vi "Handle Last Ack Core.vi"(4 "error in (no error)":errorcluster, 6 "Last Ack":refnum<class "Last Ack.lvclass">, 7 "Publisher in":refnum<class "Publisher.lvclass">) -> (0 "error out":errorcluster, 3 "Publisher out":refnum<class "Publisher.lvclass">)   [LabVIEW 2020, in "Publisher.lvlib" / "Publisher.lvclass"]
doc: "(<B>Filename</B>: Actor Framework.lvlib:Actor.lvclass:Handle Last Ack Core.vi)\n\nDefines how the caller actor responds to the Last Ack message from a nested actor. The Last Ack message is the final message a nested actor sends to its caller before it shuts down. The message contains information about the final state of the nested actor.\n\nThis implementation removes the stopped actor from the enqueuer and actor look up tables."
uses:
  Publisher.lvclass
  PPL/HDH.Actor Framework.Core.Actor.lvlibp/1abvi3w/vi.lib/ActorFramework/LastAck/Last Ack.lvclass
  Publisher.lvclass/Publisher.ctl
  PPL/HDH.Actor Framework.Core.Actor.lvlibp/1abvi3w/vi.lib/ActorFramework/Message Enqueuer/Message Enqueuer.lvclass
  PPL/HDH.Actor Framework.Core.Actor.lvlibp/1abvi3w/vi.lib/ActorFramework/Actor/Actor.lvclass
  PPL/HDH.Data.Generic.lvlibp
  PPL/HDH.Actor Framework.Core.Utility.lvlibp
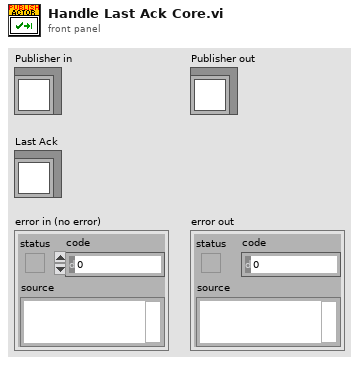
[diagram p1: front panel]
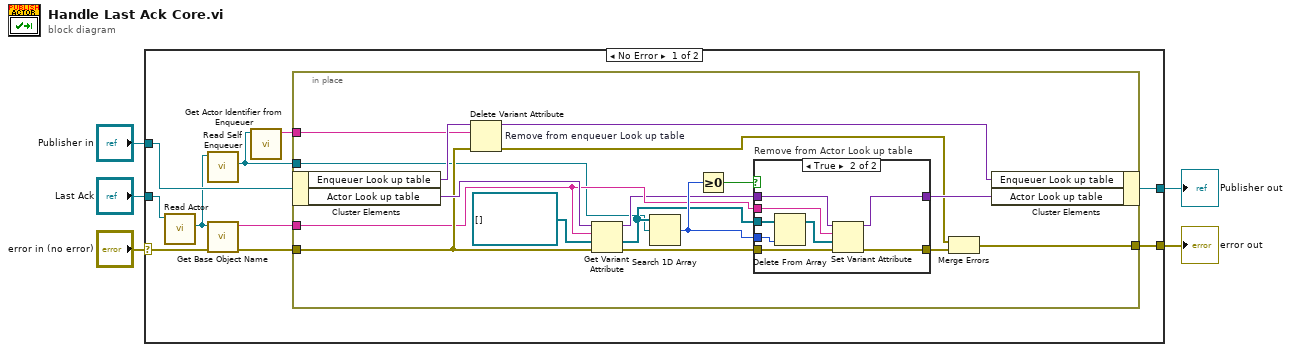
[diagram p0: block diagram]
diagram:
  n1 = case shown="No Error" "error in (no error)" {
    selector: "error in (no error)" -> [w10 w44]
    tunnel: [w8 w44] -> w4
    tunnel: [w7 w43] -> w3
    tunnel: "Publisher in" -> [w15 w43]
    tunnel: "Last Ack" -> [w13 _]
    frame No Error {
      n2 = call "Read Actor.vi"("Last Ack"=w13) -> ("Actor"=w12:refnum<class "Actor.lvclass">)  [unwired: 10 in]
      n3 = call "Read Self Enqueuer.vi"("Actor"=w12) -> ("Self Enqueuer"=w6:refnum<class "Message Enqueuer.lvclass">)  [unwired: 10 in]
      n4 = call "Get Base Object Name.vi"("error in (no error)"=w10, "Object in"=w12) -> ("error out"=w9:errorcluster, "Base class name"=w11:string)  [unwired: 8 in]
      n5 = call "Get Actor Identifier from Enqueuer.vi"("Message Enqueuer in"=w6) -> ("Actor ID string out"=w14:string)  [unwired: 9 in, 1 out]
      n6 = in-place {
        in-place-border: w14 -> [w27]
        in-place-border: w11 -> [w23]
        in-place-border: w9 -> [w28]
        in-place-border: [w17] -> w8
        in-place-border: w6 -> [w16]
        n7 = in-place-cluster #1(w15) -> ("Enqueuer Look up table"=w29:variant, "Actor Look up table"=w31:variant)
        n8 = Delete Variant Attribute "Remove from enqueuer Look up table"(4:w28, 6:w27, 7:w29) -> (0:w19:errorcluster, 3:w32:variant)  [unwired: 1 out]
        n9 = Get Variant Attribute(Variant=w31, name=w23, default value (empty Variant)=refnum<class "Message Enqueuer.lvclass">[] [] ("Message Enqueuer in"), error in=w28) -> (duplicate Variant=w22:variant, value=w24:refnum<class "Message Enqueuer.lvclass">[], error out=w20:errorcluster)  [unwired: 1 out]
        n10 = Search 1D Array(1D array=w24, element=w16) -> (index of element=w25:i32)  [unwired: 1 in]
        n11 = Greater Or Equal To 0?(x=w25) -> (x >= 0?=w26:bool)
        n12 = case "Remove from Actor Look up table" shown="True" w26 {
          tunnel: w25 -> [_ w42]
          tunnel: w24 -> [_ w41]
          tunnel: w23 -> [_ w40]
          tunnel: w22 -> [w34 w39]
          tunnel: [w34 w38] -> w21
          tunnel: w20 -> [w33 w36]
          tunnel: [w33 w35] -> w18
          frame False {
          }
          frame True {
            n13 = Delete From Array(array=w41, index=w42) -> (array with subset deleted=w37:refnum<class "Message Enqueuer.lvclass">[])  [unwired: 1 in, 1 out]
            n14 = Set Variant Attribute(Variant=w39, name=w40, value=w37, error in=w36) -> (Variant out=w38:variant, error out=w35:errorcluster)  [unwired: 1 out]
          }
        }
        n15 = Merge Errors(w19, w18) -> (w17:errorcluster)
        n16 = in-place-cluster #1("Enqueuer Look up table"=w32, "Actor Look up table"=w21) -> (w7:refnum<class "Publisher.lvclass">)
      }
    }
    frame Error {
    }
  }
  "Publisher out" <- w3
  "error out" <- w4
